vi "DG535ControlLoop.vi"(5 "Settings":T7={"Trigger"={"Trigger Mode"=enum."External", "Internal/Burst Rate"=10.0, "External  Level"=1.0, "Impedance"=TRUE, "Slope"=FALSE}, "Delays"=[{"Channel"=enum."A Output", "Sync To"=enum."T0 Output", "Delay"=0.0001526}, {"Channel"=enum."B Output", "Sync To"=enum."A Output", "Delay"=1.44e-05}, {"Channel"=enum."C Output", "Sync To"=enum."B Output", "Delay"=-2e-06}, {"Channel"=enum."D Output", "Sync To"=enum."B Output", "Delay"=8e-06}, {"Channel"=enum."Trigger Input", "Sync To"=enum."T0 Output", "Delay"=0.0}], "Output"=[{"Channel"=enum."T0 Output", "Level"=enum."TTL", "Load"=TRUE, "Polarity"=FALSE, "Amplitude"=4.0, "Offset"=0.0}, {"Channel"=enum."A Output", "Level"=enum."TTL", "Load"=TRUE, "Polarity"=FALSE, "Amplitude"=4.0, "Offset"=0.0}, {"Channel"=enum."B Output", "Level"=enum."TTL", "Load"=TRUE, "Polarity"=FALSE, "Amplitude"=4.0, "Offset"=0.0}, {"Channel"=enum."AB Output", "Level"=enum."TTL", "Load"=TRUE, "Polarity"=FALSE, "Amplitude"=4.0, "Offset"=0.0}, {"Channel"=enum."C Output", "Level"=enum."TTL", "Load"=TRUE, "Polarity"=FALSE, "Amplitude"=4.0, "Offset"=0.0}, {"Channel"=enum."D Output", "Level"=enum."TTL", "Load"=TRUE, "Polarity"=FALSE, "Amplitude"=4.0, "Offset"=0.0}, {"Channel"=enum."CD Output", "Level"=enum."TTL", "Load"=TRUE, "Polarity"=FALSE, "Amplitude"=4.0, "Offset"=0.0}]} {"Trigger"."External  Level" min=-2.56 max=2.56 format="%.2f"; "Trigger"."Internal/Burst Rate" min=0.001 max=1000000.0 format="%.3f"; "Output"."Offset" min=-3.0 max=4.0 format="%.2f"; "Output"."Amplitude" min=-3.0 max=4.0 format="%.2f"}, 8 "error in":errorcluster, 10 "queue in":refnum<queue>, 11 "VISA resource":refnum<visa-resource-name>) -> (0 "error out":errorcluster, 2 "queue out":refnum<queue>)   [LabVIEW 2013, in "SRS_DG535_Lib.lvlib"]
uses:
  <instrlib>/DG535/SRS_DG535_Lib.lvlib
  <instrlib>/DG535/Command/DG535_States.ctl
  <instrlib>/DG535/Command/Set Trigger.ctl
  <instrlib>/DG535/Command/DG535_TriggerMode.ctl
  <instrlib>/DG535/Command/Set Delay.ctl
  <instrlib>/DG535/Command/DG535_Channel.ctl
  <instrlib>/DG535/Command/Set Output.ctl
  <instrlib>/DG535/Command/DG535_Output.ctl
  <userlib>/Utility/ErrorLog_lib.lvlib
panel:
  in  "Quit":bool
  in  "SetAll":bool
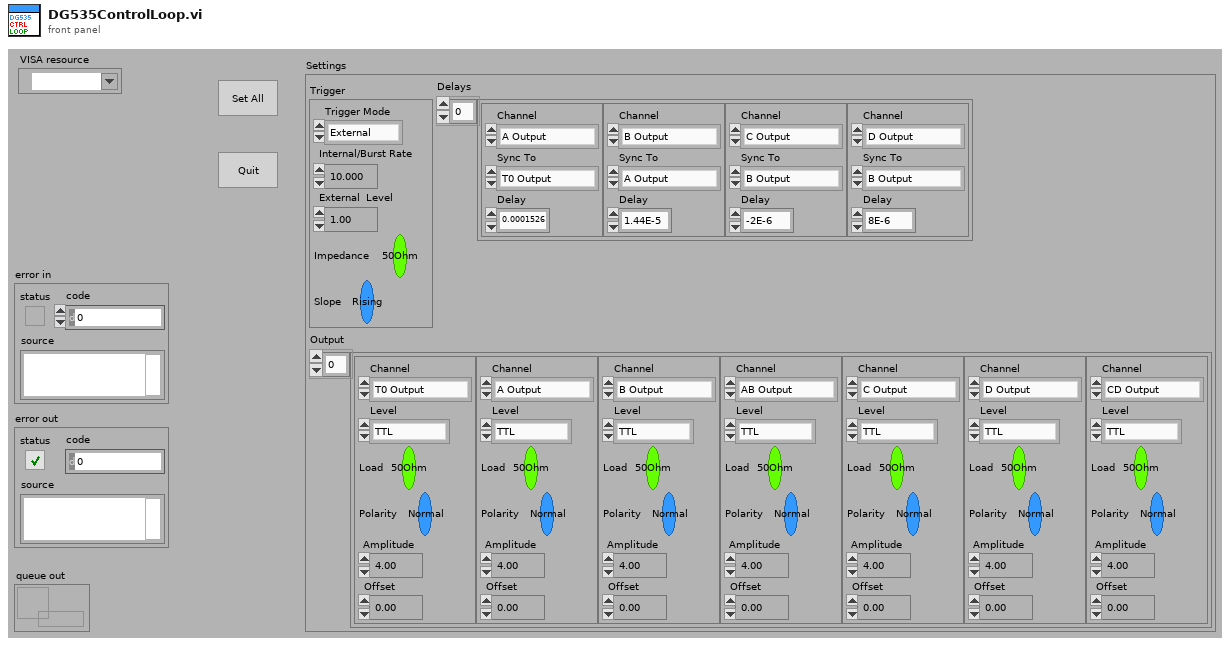
[diagram p1: front panel]
types:
  T1 = typedef "SRS_DG535_Lib.lvlib/Set Trigger.ctl" = cluster{"Trigger Mode":T2, "Internal/Burst Rate":dbl, "External  Level":sgl, "Impedance":bool, "Slope":bool}
  T2 = typedef "SRS_DG535_Lib.lvlib/DG535_TriggerMode.ctl" = enum16{"Internal", "External", "SingleShot", "Burst", "Line"}
  T3 = typedef "SRS_DG535_Lib.lvlib/Set Delay.ctl" = cluster{"Channel":T4, "Sync To":T4, "Delay":dbl}
  T4 = typedef "SRS_DG535_Lib.lvlib/DG535_Channel.ctl" = enum16{"Trigger Input", "T0 Output", "A Output", "B Output", "AB Output", "C Output", "D Output", "CD Output", "NULL"}
  T5 = typedef "SRS_DG535_Lib.lvlib/Set Output.ctl" = cluster{"Channel":T4, "Level":T6, "Load":bool, "Polarity":bool, "Amplitude":dbl, "Offset":dbl}
  T6 = typedef "SRS_DG535_Lib.lvlib/DG535_Output.ctl" = enum16{"TTL", "NIM", "ECL", "Variable"}
  T7 = cluster{"Trigger":T1, "Delays":T3[], "Output":T5[]}
  T8 = typedef "SRS_DG535_Lib.lvlib/DG535_States.ctl" = cluster{"State":enum16{"Initialize", "Set Trigger", "Set Output", "Set Delay", "Manl_Trig", "Run", "Stop", "Close", "Quit"}, "Para.":variant}
  T9 = enum16{"Initialize", "Set Trigger", "Set Output", "Set Delay", "Manl_Trig", "Run", "Stop", "Close", "Quit"}
  T10 = cluster{"Baud Rate":u32, "Parity":u16, "Data Bits":u16, "Stop Bits":u16, "Flow Control":u16}
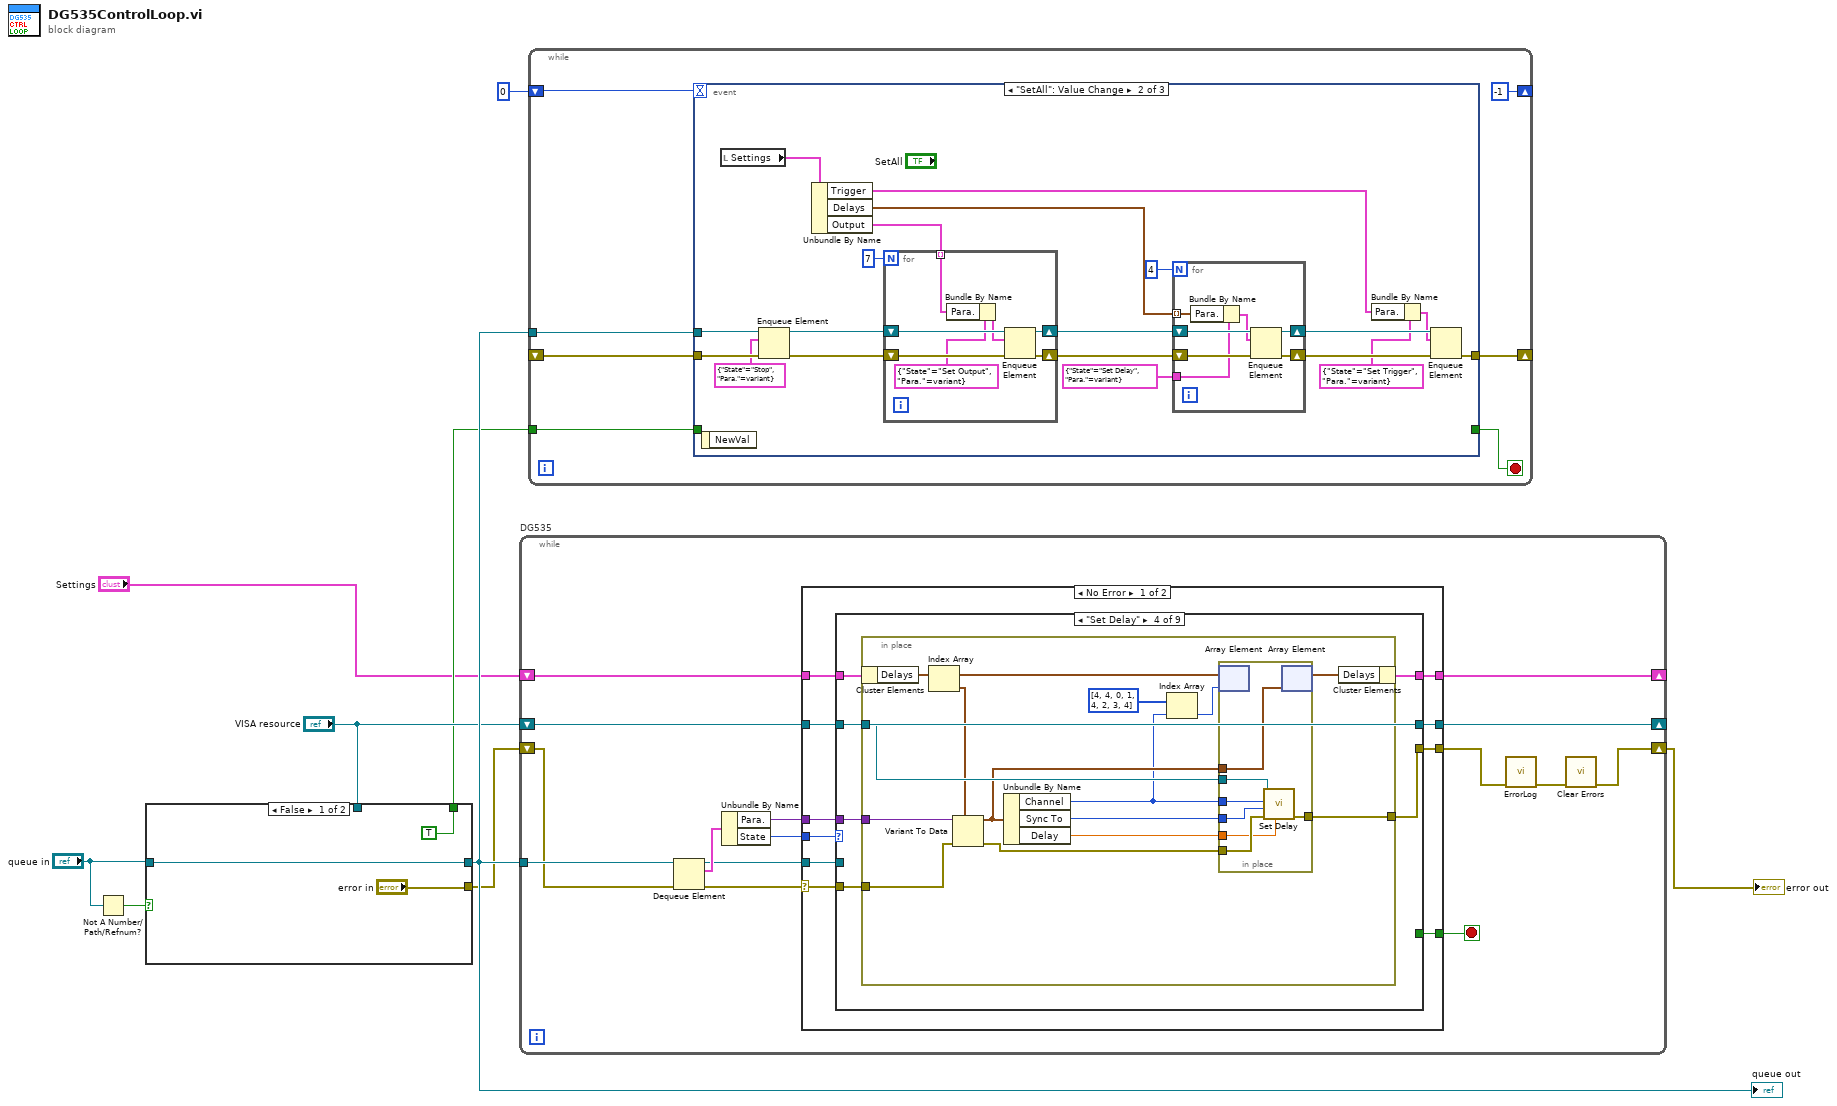
[diagram p0: block diagram]
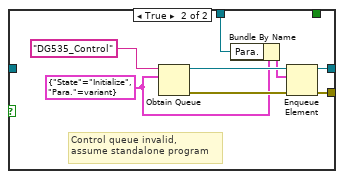
[diagram p2: hidden frame]
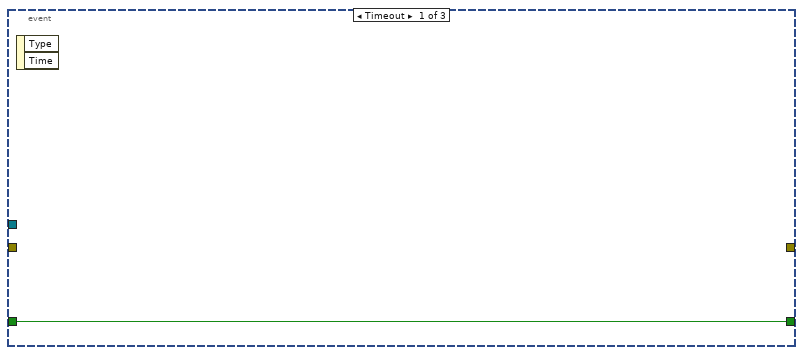
[diagram p3: hidden frame]
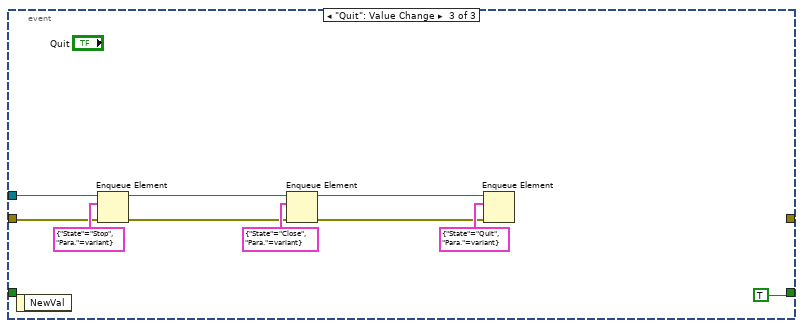
[diagram p4: hidden frame]
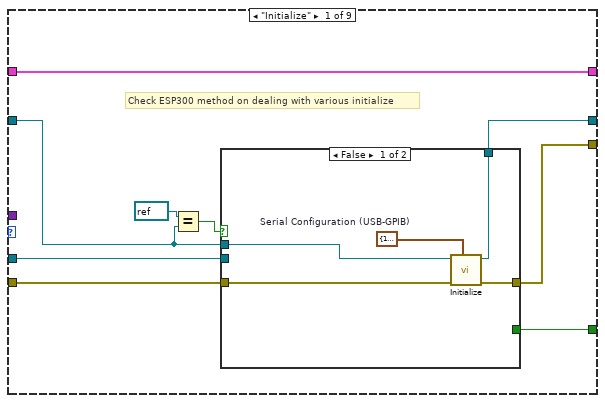
[diagram p5: hidden frame]
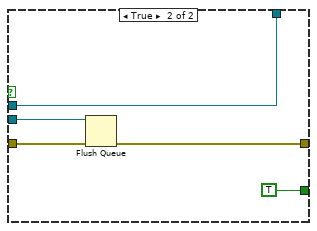
[diagram p6: hidden frame]
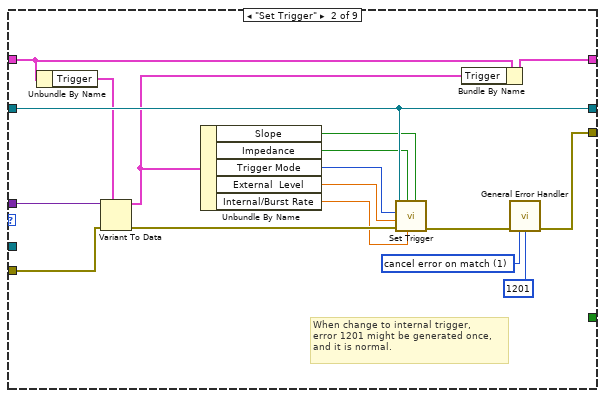
[diagram p7: hidden frame]
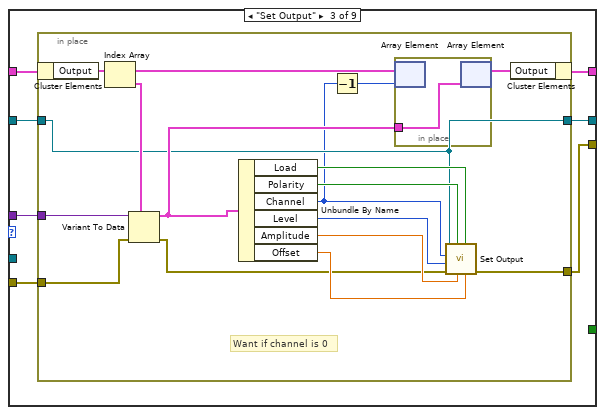
[diagram p8: hidden frame]
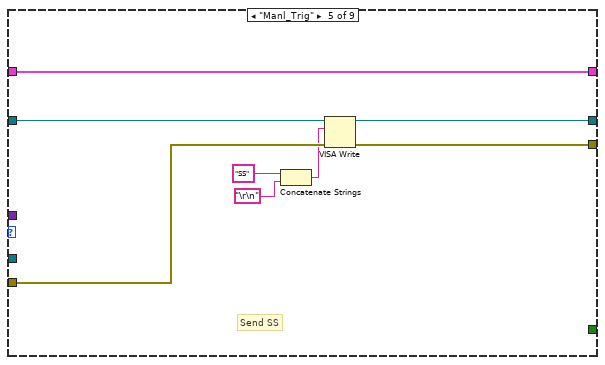
[diagram p9: hidden frame]
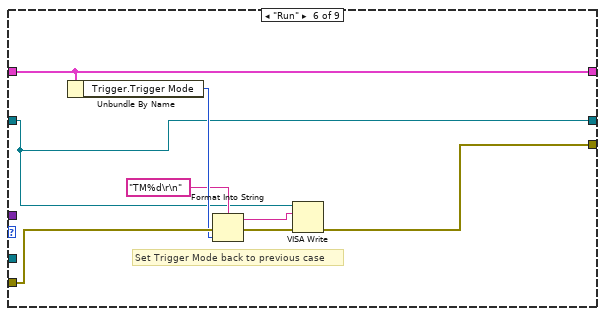
[diagram p10: hidden frame]
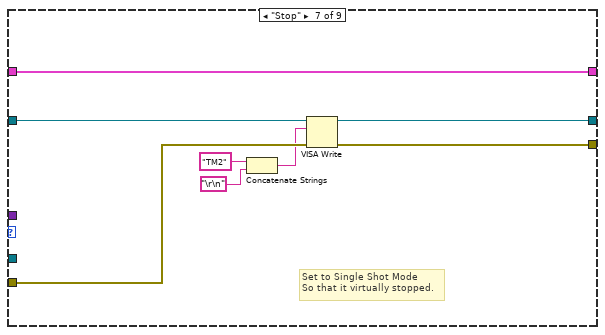
[diagram p11: hidden frame]
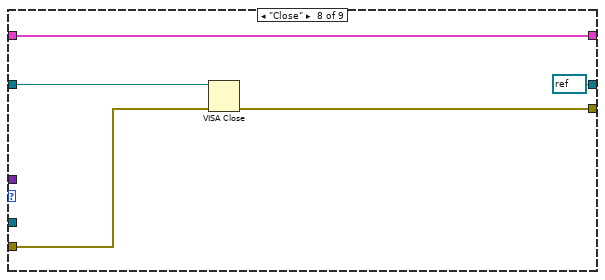
[diagram p12: hidden frame]
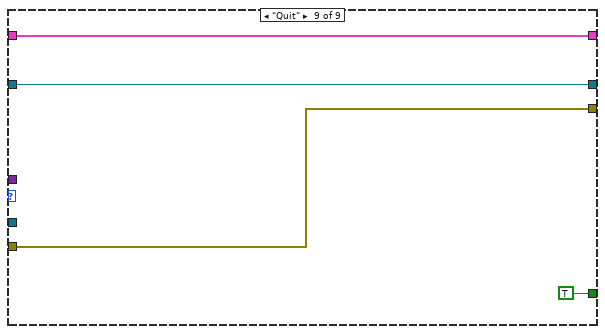
[diagram p13: hidden frame]
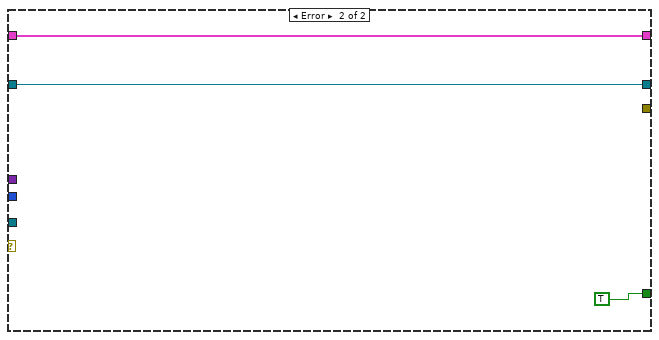
[diagram p14: hidden frame]
diagram:
  n1 = Not A Number/Path/Refnum?(number/path/refnum="queue in") -> (NaN/Path/Refnum?=w8:bool)
  n2 = case shown="False" w8 {
    tunnel: [w12 w17] -> w7
    tunnel: ["error in" w19] -> w5
    tunnel: "queue in" -> [w12 _]
    tunnel: "VISA resource" -> [_ w13]
    tunnel: [TRUE _] -> w3
    frame False {
    }
    frame True {
      w15 = T8 {"State"=enum."Initialize", "Para."=variant} ("element")
      # "Control queue invalid, \nassume standalone program"
      n3 = Obtain Queue(name (unnamed)="DG535_Control", element data type=w15) -> (queue out=w18:refnum<queue>, error out=w19:errorcluster)  [unwired: 3 in, 1 out]
      n4 = Bundle By Name(cluster=w15, "Para."=w13) -> (w14:T8)
      n5 = Enqueue Element(queue=w18, element=w14) -> (queue out=w17:refnum<queue>)  [unwired: 2 in, 2 out]
    }
  }
  "queue out" <- w7
  n6 = while "DG535" {
    tunnel: w7 -> [w34]
    shift-right: [w22] -> w9
    shift-left: w5 -> [w23]
    shift-right: [w25] -> _
    shift-left: "Settings" -> [w26]
    shift-right: [w24] -> _
    shift-left: "VISA resource" -> [w29]
    stop <- w27 stop-if-true
    n7 = Dequeue Element(queue=w34, error in (no error)=w23) -> (queue out=w30:refnum<queue>, element=w33:T8, error out=w28:errorcluster)  [unwired: 1 in, 1 out]
    n8 = Unbundle By Name(w33) -> ("Para."=w31:variant, "State"=w32:T9)
    n9 = case shown="No Error" w28 {
      selector: w28 -> [w36 _]
      tunnel: w32 -> [w44 _]
      tunnel: w31 -> [w43 _]
      tunnel: w30 -> [w42 _]
      tunnel: w29 -> [w41 w165]
      tunnel: [w40 _] -> w20
      tunnel: [w35 TRUE] -> w27
      tunnel: w26 -> [w39 w166]
      tunnel: [w38 w166] -> w25
      tunnel: [w37 w165] -> w24
      frame No Error {
        n10 = case shown="\"Set Delay\"" w44 {
          tunnel: w43 -> [_ w80 w85 w110 _ _ _ _ _]
          tunnel: w42 -> [w45 _ _ _ _ _ _ _ _]
          tunnel: w41 -> [w48 w78 w86 w109 w136 w140 w151 w159 w162]
          tunnel: w36 -> [w52 w76 w84 w107 w138 w145 w154 w156 w164]
          tunnel: [w51 w64 w81 w108 w137 w147 w153 w158 w164] -> w40
          tunnel: w39 -> [w53 w74 w87 w106 w139 w144 w155 w160 w163]
          tunnel: [w53 w77 w82 w105 w139 w144 w155 w160 w163] -> w38
          tunnel: [w50 w78 w83 w109 w135 w140 w150 refnum<visa-resource-name> refnum ("VISA resource") w162] -> w37
          tunnel: [w46 _ _ _ _ _ _ _ TRUE] -> w35
          frame "Initialize" {
            # "Check ESP300 method on dealing with various initialize"
            n11 = Equal?(x=refnum<visa-resource-name> refnum ("VISA resource"), y=w48) -> (x = y?=w49:bool)
            n12 = case shown="False" w49 {
              tunnel: w52 -> [w58 w63]
              tunnel: w48 -> [w57 w61]
              tunnel: [w56 w60] -> w51
              tunnel: [w55 w61] -> w50
              tunnel: [_ TRUE] -> w46
              tunnel: w45 -> [_ w59]
              frame False {
                w54 = T10 {"Baud Rate"=115200, "Parity"=0, "Data Bits"=8, "Stop Bits"=10, "Flow Control"=0}  # Serial Configuration (USB-GPIB)
                n13 = call <instrlib>:"Initialize.vi"("Serial Configuration"=w54, "error in (no error)"=w58, "VISA resource name"=w57) -> ("error out"=w56:errorcluster, "VISA resource name out"=w55:refnum<visa-resource-name>)  [unwired: 7 in]
              }
              frame True {
                n14 = Flush Queue(queue=w59, error in (no error)=w63) -> (error out=w60:errorcluster)  [unwired: 2 out]
              }
            }
          }
          frame "Set Trigger" {
            w67 = 1 items=["no exception", "cancel error on match", "set error on match"] ("[exception action] (none:0)")
            # "When change to internal trigger,\nerror 1201 might be generated once, \nand it is normal."
            n15 = Unbundle By Name(w74) -> ("Trigger"=w73:T1)
            n16 = Variant To Data(error in=w76, type=w73, Variant=w80) -> (data=w72:T1, error out=w79:errorcluster)
            n17 = Unbundle By Name(w72) -> ("Slope"=w75:bool, "Impedance"=w69:bool, "Trigger Mode"=w71:T2, "External  Level"=w68:sgl, "Internal/Burst Rate"=w70:dbl)
            n18 = call <instrlib>:"Set Trigger.vi"("Trigger Slope"=w75, "internal/burst trigger rate"=w70, "Input Impedance"=w69, "error in (no error)"=w79, "external trigger level"=w68, "Trigger Mode"=w71, "VISA Refnum in"=w78) -> ("error out"=w65:errorcluster)  [unwired: 4 in]
            n19 = Bundle By Name(cluster=w74, "Trigger"=w72) -> (w77:T7)
            n20 = call <vilib>:"General Error Handler.vi"("error in (no error)"=w65, "[exception action] (none:0)"=w67, "[exception code]"=1201) -> ("error out"=w64:errorcluster)  [unwired: 8 in, 4 out]
          }
          frame "Set Output" {
            n21 = in-place {
              in-place-border: w85 -> [w103]
              in-place-border: w86 -> [w90]
              in-place-border: w84 -> [w102]
              in-place-border: [w91] -> w81
              in-place-border: [w90] -> w83
              # "Want if channel is 0"
              n22 = in-place-cluster #1(w87) -> ("Output"=w100:T5[])
              n23 = Index Array(array=w100) -> (element=w101:T5)  [unwired: 1 in]
              n24 = Variant To Data(error in=w102, type=w101, Variant=w103) -> (data=w93:T5, error out=w92:errorcluster)
              n25 = Unbundle By Name(w93) -> ("Load"=w94:bool, "Polarity"=w95:bool, "Channel"=w89:T4, "Level"=w98:T6, "Amplitude"=w97:dbl, "Offset"=w96:dbl)
              n26 = Decrement(x=w89) -> (x-1=w88:T4)
              n27 = in-place {
                in-place-border: w93 -> [w104]
                n28 = in-place-array #2(w100, w88) -> ()  [unwired: 1 out]
                n29 = in-place-array #2(w104) -> (w99:T5[])  [unwired: 1 out]
              }
              n30 = call <instrlib>:"Set Output.vi"("Offset"=w96, "Load"=w94, "Amplitude"=w97, "Polarity"=w95, "error in (no error)"=w92, "Output Level"=w98, "Channel"=w89, "VISA Refnum in"=w90) -> ("error out"=w91:errorcluster)  [unwired: 3 in]
              n31 = in-place-cluster #1("Output"=w99) -> (w82:T7)
            }
          }
          frame "Set Delay" {
            n32 = in-place {
              in-place-border: w110 -> [w124]
              in-place-border: w109 -> [w123]
              in-place-border: [w122] -> w108
              in-place-border: w107 -> [w121]
              n33 = in-place-cluster #3(w106) -> ("Delays"=w116:T3[])
              n34 = Index Array(array=w116) -> (element=w117:T3)  [unwired: 1 in]
              n35 = Variant To Data(error in=w121, type=w117, Variant=w124) -> (data=w115:T3, error out=w120:errorcluster)
              n36 = Unbundle By Name(w115) -> ("Channel"=w112:T4, "Sync To"=w119:T4, "Delay"=w118:dbl)
              n37 = Index Array(array=i32[] [4, 4, 0, 1, 4, 2, 3, 4], index=w112) -> (element=w111:i32)
              n38 = in-place {
                in-place-border: w123 -> [w131]
                in-place-border: [w130] -> w122
                in-place-border: w120 -> [w129]
                in-place-border: w112 -> [w128]
                in-place-border: w119 -> [w127]
                in-place-border: w118 -> [w126]
                in-place-border: w115 -> [w125]
                n39 = in-place-array #4(w116, w111) -> ()  [unwired: 1 out]
                n40 = call <instrlib>:"Set Delay.vi"("Delay (s)"=w126, "error in (no error)"=w129, "Sync To"=w127, "Channel"=w128, "VISA Refnum in"=w131) -> ("error out"=w130:errorcluster)  [unwired: 6 in]
                n41 = in-place-array #4(w125) -> (w114:T3[])  [unwired: 1 out]
              }
              n42 = in-place-cluster #3("Delays"=w114) -> (w105:T7)
            }
          }
          frame "Manl_Trig" {
            # "Send SS"
            n43 = Concatenate Strings("SS" ("write buffer"), "\r\n") -> (w133:string)
            n44 = VISA Write(VISA resource name=w136, write buffer=w133, error in (no error)=w138) -> (VISA resource name out=w135:refnum<visa-resource-name>, error out=w137:errorcluster)  [unwired: 1 out]
          }
          frame "Run" {
            # "Set Trigger Mode back to previous case"
            n45 = Unbundle By Name(w144) -> ("Trigger.Trigger Mode"=w143:T2)
            n46 = Format Into String(format string="TM%d\r\n", error in=w145, w143) -> (resulting string=w141:string, error out=w146:errorcluster)  [unwired: 1 in]
            n47 = VISA Write(VISA resource name=w140, write buffer=w141, error in (no error)=w146) -> (error out=w147:errorcluster)  [unwired: 2 out]
          }
          frame "Stop" {
            # "Set to Single Shot Mode\nSo that it virtually stopped."
            n48 = Concatenate Strings("TM2" ("write buffer"), "\r\n") -> (w149:string)
            n49 = VISA Write(VISA resource name=w151, write buffer=w149, error in (no error)=w154) -> (VISA resource name out=w150:refnum<visa-resource-name>, error out=w153:errorcluster)  [unwired: 1 out]
          }
          frame "Close" {
            n50 = VISA Close(VISA resource name=w159, error in (no error)=w156) -> (error out=w158:errorcluster)
          }
          frame "Quit" {
          }
        }
      }
      frame Error {
      }
    }
    n51 = call <userlib>:"ErrorLog.vi"("error in (no error)"=w20) -> ("error out"=w21:errorcluster)  [unwired: 10 in]
    n52 = call <vilib>:"Clear Errors.vi"("error in (no error)"=w21) -> ("error out"=w22:errorcluster)  [unwired: 6 in]
  }
  "error out" <- w9
  n53 = while {
    tunnel: w7 -> [w174]
    shift-right: [w173] -> _
    shift-left: _ -> [w172]
    tunnel: w3 -> [w170]
    shift-right: [-1] -> _
    shift-left: 0 -> [w169]
    stop <- w171 stop-if-true
    n54 = event shown="[1] \"SetAll\": Value Change" {
      selector: _ -> [_ _ _]
      dyn-events: _ -> [_ _ _]
      timeout: w169 -> [_ _ _]
      tunnel: w174 -> [_ w194 w215]
      tunnel: [_ w182 _] -> w173
      tunnel: w172 -> [_ w188 w216]
      tunnel: [w175 _ TRUE] -> w171
      tunnel: w170 -> [w175 _ _]
      event Timeout {
        n55 = event-data() -> ()  [unwired: 1 in, 2 out]
      }
      event "SetAll": Value Change {
        n56 = event-data() -> ()  [unwired: 1 in, 1 out]
        n57 = local read "Settings"() -> (w176:T7)
        n58 = Enqueue Element(queue=w194, element=T8 {"State"=enum."Stop", "Para."=variant}, error in (no error)=w188) -> (queue out=w193:refnum<queue>, error out=w190:errorcluster)  [unwired: 1 in, 1 out]
        n59 = Unbundle By Name(w176) -> ("Trigger"=w179:T1, "Delays"=w185:T3[], "Output"=w178:T5[])
        n60 = for {
          N: 7 -> [_]
          shift-right: [w200] -> w192
          shift-left: w193 -> [w201]
          shift-right: [w198] -> w189
          shift-left: w190 -> [w199]
          tunnel: w178 -> [w195] mode=indexing
          n61 = Bundle By Name(cluster=T8 {"State"=enum."Set Output", "Para."=variant} ("element"), "Para."=w195) -> (w196:T8)
          n62 = Enqueue Element(queue=w201, element=w196, error in (no error)=w199) -> (queue out=w200:refnum<queue>, error out=w198:errorcluster)  [unwired: 1 in, 1 out]
        }
        n63 = for {
          N: 4 -> [_]
          shift-right: [w206] -> w183
          shift-left: w189 -> [w207]
          tunnel: T8 {"State"=enum."Set Delay", "Para."=variant} ("element") -> [w205]
          tunnel: w185 -> [w203] mode=indexing
          shift-right: [w202] -> w184
          shift-left: w192 -> [w208]
          n64 = Bundle By Name(cluster=w205, "Para."=w203) -> (w204:T8)
          n65 = Enqueue Element(queue=w208, element=w204, error in (no error)=w207) -> (queue out=w202:refnum<queue>, error out=w206:errorcluster)  [unwired: 1 in, 1 out]
        }
        n66 = Bundle By Name(cluster=T8 {"State"=enum."Set Trigger", "Para."=variant} ("element"), "Para."=w179) -> (w180:T8)
        n67 = Enqueue Element(queue=w184, element=w180, error in (no error)=w183) -> (error out=w182:errorcluster)  [unwired: 1 in, 2 out]
      }
      event "Quit": Value Change {
        n68 = event-data() -> ()  [unwired: 1 in, 1 out]
        n69 = Enqueue Element(queue=w215, element=T8 {"State"=enum."Stop", "Para."=variant}, error in (no error)=w216) -> (queue out=w210:refnum<queue>, error out=w209:errorcluster)  [unwired: 1 in, 1 out]
        n70 = Enqueue Element(queue=w210, element=T8 {"State"=enum."Close", "Para."=variant}, error in (no error)=w209) -> (queue out=w212:refnum<queue>, error out=w211:errorcluster)  [unwired: 1 in, 1 out]
        n71 = Enqueue Element(queue=w212, element=T8 {"State"=enum."Quit", "Para."=variant}, error in (no error)=w211) -> ()  [unwired: 1 in, 3 out]
      }
    }
  }
